vi "AB_RESTfulVI_Configuration_Dialog.vi"(8 "error in (no error)":errorcluster, 11 "RESTful VI configuration in":T1={"Service VI Type"=enum."Web Method", "Load VI at statup"=TRUE, "Keep VI in memory"=TRUE, "Output type"=enum."Terminal", "Output format"=enum."XML", "Use headers"=TRUE, "Buffered"=TRUE, "eng_Load VI by name"=FALSE}) -> (0 "error out":errorcluster, 2 "cancelled?":bool, 3 "RESTful VI configuration out":T1={"Service VI Type"=enum."Web Method", "Load VI at statup"=TRUE, "Keep VI in memory"=TRUE, "Output type"=enum."Terminal", "Output format"=enum."XML", "Use headers"=TRUE, "Buffered"=TRUE, "eng_Load VI by name"=FALSE})   [LabVIEW 2020]
uses:
  <vilib>/AppBuilder/AB_Classes/Source/RESTfulVI/Configure_RESTfulVI/AB_RESTful_Configuration.ctl
  <vilib>/AppBuilder/AB_Classes/Source/RESTfulVI/Configure_RESTfulVI/AB_RESTful_VIType.ctl
  <vilib>/AppBuilder/AB_Classes/Source/RESTfulVI/Configure_RESTfulVI/AB_RESTful_OutputType.ctl
  <vilib>/AppBuilder/AB_Classes/Source/RESTfulVI/Configure_RESTfulVI/AB_RESTful_OutputFormat.ctl
panel:
  in  "Keep VI in memory":bool=TRUE
  in  "Load VI at statup":bool=TRUE
  in  "Output format":u16(ring) items=["XML", "Text", "HTML", "JSON"]
  in  "Buffered":bool=TRUE
  in  "Use headers":bool=TRUE
  in  "Output type":enum32{"Terminal", "Stream"}(radio)
  in  "Service VI Type":enum32{"Web Method", "Auxiliary"}(radio)
  in  "Help":bool
  in  "Cancel":bool
  in  "OK":bool
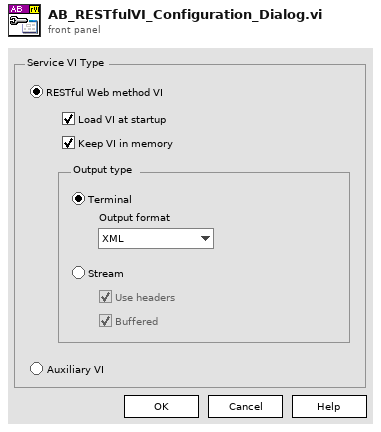
[diagram p1: front panel]
types:
  T1 = typedef "AB_RESTful_Configuration.ctl" = cluster{"Service VI Type":T2, "Load VI at statup":bool, "Keep VI in memory":bool, "Output type":T3, "Output format":T4, "Use headers":bool, "Buffered":bool, "eng_Load VI by name":bool}
  T2 = typedef "AB_RESTful_VIType.ctl" = enum32{"Web Method", "Auxiliary", "eng_Internal", "eng_Content"}
  T3 = typedef "AB_RESTful_OutputType.ctl" = enum32{"Terminal", "Stream"}
  T4 = typedef "AB_RESTful_OutputFormat.ctl" = enum32{"XML", "Text", "HTML", "JSON"}
  T5 = enum32{"Invalid", "Standard", "Closed", "Hidden", "Minimized", "Maximized"}
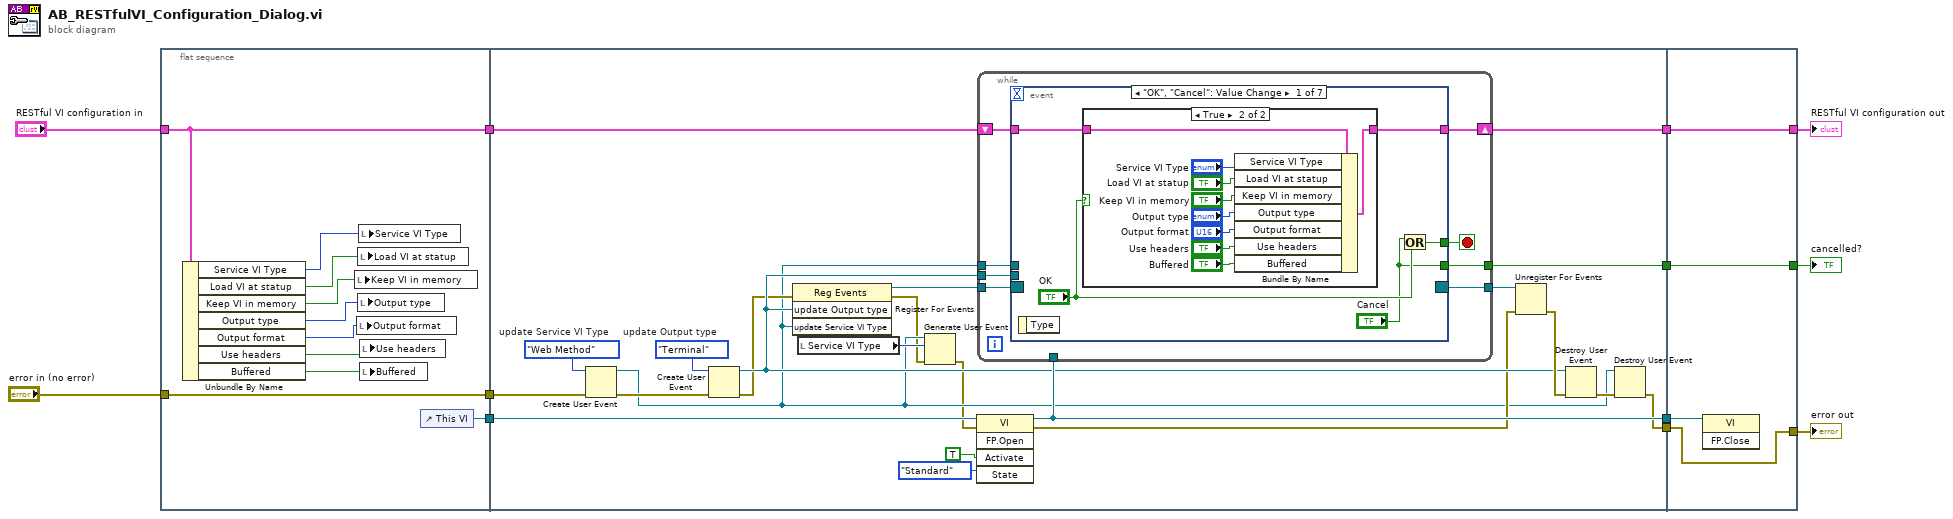
[diagram p0: block diagram]
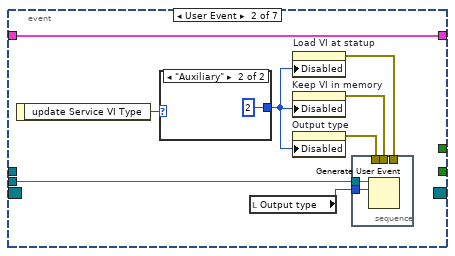
[diagram p3: hidden frame]
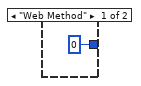
[diagram p4: hidden frame]
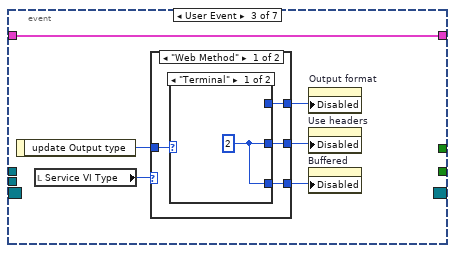
[diagram p5: hidden frame]
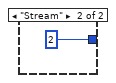
[diagram p6: hidden frame]
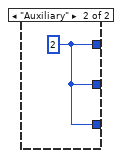
[diagram p7: hidden frame]
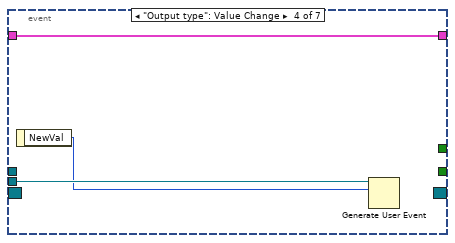
[diagram p8: hidden frame]
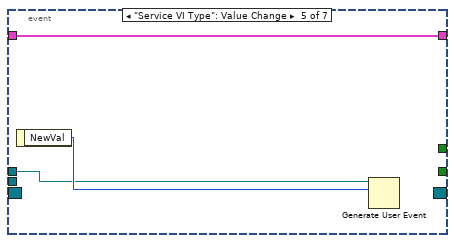
[diagram p9: hidden frame]
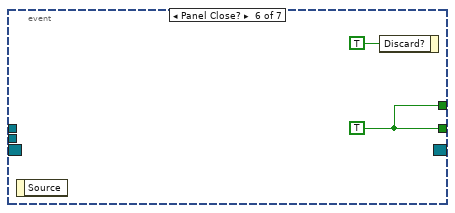
[diagram p10: hidden frame]
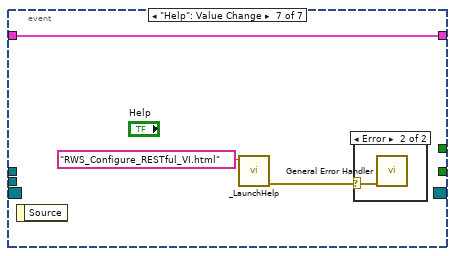
[diagram p11: hidden frame]
diagram:
  n1 = flat-sequence {
    tunnel: [w22] -> w12
    tunnel: "RESTful VI configuration in" -> [w20]
    tunnel: [w20] -> w5
    tunnel: "error in (no error)" -> [w21]
    tunnel: [w21] -> w1
    tunnel: w12 -> [w43]
    tunnel: [w42] -> w11
    tunnel: [w31] -> w10
    tunnel: [w41] -> w9
    tunnel: w5 -> [w25]
    tunnel: [w24] -> w4
    tunnel: w1 -> [w23]
    tunnel: w11 -> [w108]
    tunnel: w10 -> [w107]
    tunnel: [w107] -> w7
    tunnel: w9 -> [w106]
    tunnel: [w106] -> w8
    tunnel: w4 -> [w105]
    tunnel: [w105] -> w3
    frame #0 {
      n2 = Unbundle By Name(w20) -> ("Service VI Type"=w13:T2, "Load VI at statup"=w19:bool, "Keep VI in memory"=w18:bool, "Output type"=w17:T3, "Output format"=w14:T4, "Use headers"=w16:bool, "Buffered"=w15:bool)
      n3 = local write "Keep VI in memory"(w18) -> ()
      n4 = local write "Output format"(w14) -> ()
      n5 = local write "Load VI at statup"(w19) -> ()
      n6 = local write "Output type"(w17) -> ()
      n7 = local write "Service VI Type"(w13) -> ()
      n8 = local write "Use headers"(w16) -> ()
      n9 = local write "Buffered"(w15) -> ()
      n10 = control-ref of="This VI"() -> (w22:refnum<vi>)
    }
    frame #1 {
      w34 = enum32{"Web Method", "Auxiliary"}."Web Method"  # update Service VI Type
      w37 = enum32{"Terminal", "Stream"}."Terminal"  # update Output type
      n11 = Create User Event(user event datatype=w34, error in=w23) -> (user event=w28:refnum<user-event>, error out=w29:errorcluster)
      n12 = Create User Event(user event datatype=w37, error in=w29) -> (user event=w36:refnum<user-event>, error out=w35:errorcluster)
      n13 = register-events(error in=w35, w36, w28) -> (reference out=w40:refnum<event-registration>, error out=w26:errorcluster)  [unwired: 1 in]
      n14 = local read "Service VI Type"() -> (w30:enum32{"Web Method", "Auxiliary"})
      n15 = Generate User Event(user event=w28, event data cluster=w30, error in=w26) -> (error out=w27:errorcluster)  [unwired: 1 in, 1 out]
      n16 = invoke class="VI" method="FP.Open"(reference=w43, error in=w27, "Activate"=TRUE, "State"=T5."Standard") -> (reference out=w42:refnum<vi>, error out=w33:errorcluster)  [unwired: 1 in, 3 out]
      n17 = while {
        tunnel: w42 -> [_]
        tunnel: [w52] -> w41
        tunnel: w40 -> [w51]
        tunnel: [w50] -> w39
        tunnel: w36 -> [w49]
        tunnel: w28 -> [w48]
        shift-right: [w46] -> w24
        shift-left: w25 -> [w47]
        stop <- w53 stop-if-true
        n18 = event shown="[0] \"OK\", \"Cancel\": Value Change" {
          selector: w51 -> [_ _ _ _ _ _ _]
          dyn-events: [_ _ _ _ _ _ _] -> w50
          timeout: _ -> [_ _ _ _ _ _ _]
          tunnel: [w58 _ _ _ _ w99 _] -> w53
          tunnel: ["Cancel" _ _ _ _ w99 _] -> w52
          tunnel: w49 -> [_ w73 _ w95 _ _ _]
          tunnel: w48 -> [_ _ _ _ w97 _ _]
          tunnel: w47 -> [w57 w68 w80 w93 w96 _ w101]
          tunnel: [w56 w68 w80 w93 w96 _ w101] -> w46
          event "OK", "Cancel": Value Change {
            n19 = event-data() -> ()  [unwired: 2 out]
            n20 = case shown="True" "OK" {
              tunnel: w57 -> [_ w67]
              tunnel: [_ w66] -> w56
              frame False {
              }
              frame True {
                n21 = Bundle By Name(cluster=w67, "Service VI Type"="Service VI Type", "Load VI at statup"="Load VI at statup", "Keep VI in memory"="Keep VI in memory", "Output type"="Output type", "Output format"="Output format", "Use headers"="Use headers", "Buffered"="Buffered") -> (w66:T1)
              }
            }
            n22 = Or(x="Cancel", y="OK") -> (x .or. y?=w58:bool)
          }
          event User Event {
            n23 = event-data() -> ("update Service VI Type"=w75:enum32{"Web Method", "Auxiliary"})  [unwired: 1 out]
            n24 = case shown="\"Auxiliary\"" w75 {
              tunnel: [u8 0 ("Disabled") u8 2 ("Disabled")] -> w74
              frame "Web Method" {
              }
              frame "Auxiliary" {
              }
            }
            n25 = local read "Output type"() -> (w72:enum32{"Terminal", "Stream"})
            n26 = property on="Load VI at statup" class="Bool (strict)"("Disabled"=w74) -> (error out=w69:errorcluster)  [unwired: 2 in, 1 out]
            n27 = property on="Keep VI in memory" class="Bool (strict)"("Disabled"=w74) -> (error out=w70:errorcluster)  [unwired: 2 in, 1 out]
            n28 = property on="Output type" class="RadioBtnsControl (strict)"("Disabled"=w74) -> (error out=w71:errorcluster)  [unwired: 2 in, 1 out]
            n29 = stacked-sequence {
              tunnel: w73 -> [w77]
              tunnel: w72 -> [w76]
              tunnel: w71 -> [_]
              tunnel: w70 -> [_]
              tunnel: w69 -> [_]
              frame #0 {
                n30 = Generate User Event(user event=w77, event data cluster=w76) -> ()  [unwired: 2 in, 2 out]
              }
            }
          }
          event User Event {
            n31 = event-data() -> ("update Output type"=w85:enum32{"Terminal", "Stream"})  [unwired: 1 out]
            n32 = local read "Service VI Type"() -> (w81:enum32{"Web Method", "Auxiliary"})
            n33 = case shown="\"Web Method\"" w81 {
              tunnel: w85 -> [w89 _]
              tunnel: [w88 w92] -> w84
              tunnel: [w87 w92] -> w83
              tunnel: [w86 w92] -> w82
              frame "Web Method" {
                n34 = case shown="\"Terminal\"" w89 {
                  tunnel: [_ u8 2 ("Disabled")] -> w88
                  tunnel: [w90 _] -> w87
                  tunnel: [w90 _] -> w86
                  frame "Terminal" {
                    w90 = u8 2 ("Disabled")
                  }
                  frame "Stream" {
                  }
                }
              }
              frame "Auxiliary" {
                w92 = u8 2 ("Disabled")
              }
            }
            n35 = property on="Output format" class="Ring (strict)"("Disabled"=w84) -> ()  [unwired: 2 in, 2 out]
            n36 = property on="Use headers" class="Bool (strict)"("Disabled"=w83) -> ()  [unwired: 2 in, 2 out]
            n37 = property on="Buffered" class="Bool (strict)"("Disabled"=w82) -> ()  [unwired: 2 in, 2 out]
          }
          event "Output type": Value Change {
            n38 = event-data() -> ("NewVal"=w94:enum32{"Terminal", "Stream"})  [unwired: 1 out]
            n39 = Generate User Event(user event=w95, event data cluster=w94) -> ()  [unwired: 2 in, 2 out]
          }
          event "Service VI Type": Value Change {
            n40 = event-data() -> ("NewVal"=w98:enum32{"Web Method", "Auxiliary"})  [unwired: 1 out]
            n41 = Generate User Event(user event=w97, event data cluster=w98) -> ()  [unwired: 2 in, 2 out]
          }
          event Panel Close? {
            w99 = TRUE ("Cancel")
            n42 = event-data() -> ()  [unwired: 2 out]
            n43 = event-data("Discard?"=TRUE) -> ()  [unwired: 1 in, 1 out]
          }
          event "Help": Value Change {
            n44 = event-data() -> ()  [unwired: 2 out]
            n45 = call <helpdir>:"_LaunchHelp.vi"("HTML filename"="RWS_Configure_RESTful_VI.html") -> ("error out"=w103:errorcluster)  [unwired: 2 in, 4 out]
            n46 = case shown="Error" w103 {
              selector: w103 -> [_ w104]
              frame No Error {
              }
              frame Error {
                n47 = call <vilib>:"General Error Handler.vi"("error in (no error)"=w104) -> ()  [unwired: 2 in, 13 out]
              }
            }
          }
        }
      }
      n48 = Unregister For Events(event registration refnum=w39, error in=w33) -> (error out=w38:errorcluster)
      n49 = Destroy User Event(user event=w36, error in=w38) -> (error out=w32:errorcluster)
      n50 = Destroy User Event(user event=w28, error in=w32) -> (error out=w31:errorcluster)
    }
    frame #2 {
      n51 = invoke class="VI" method="FP.Close"(reference=w108) -> ()  [unwired: 2 in, 3 out]
    }
  }
  "cancelled?" <- w8
  "error out" <- w7
  "RESTful VI configuration out" <- w3
